vi "Write WriteUrgent.vi"(8 "error in (no error)":errorcluster, 10 "WriteUrgent":refnum<notifier>, 11 "ICPCON ET Data Model in":refnum<class "ICPCON ET Data Model.lvclass">) -> (0 "error out":errorcluster, 3 "ICPCON ET Data Model out":refnum<class "ICPCON ET Data Model.lvclass">)   [LabVIEW 2021, in "ICPCON ET Data Model.lvclass"]
uses:
  ICPCON ET Data Model.lvclass
  ICPCON ET Data Model.lvclass/ICPCON ET Data Model.ctl
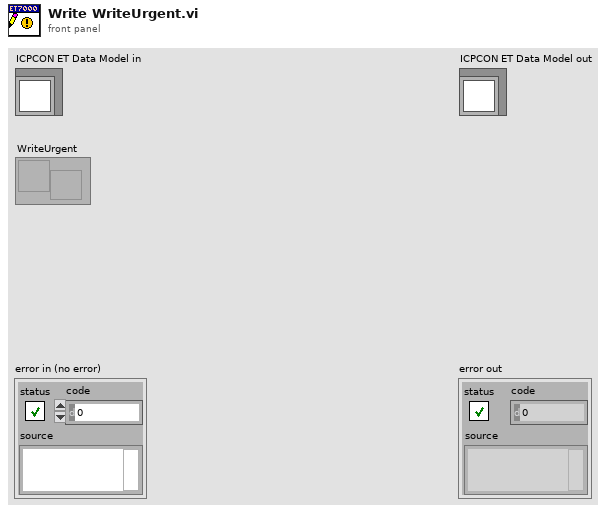
[diagram p1: front panel]
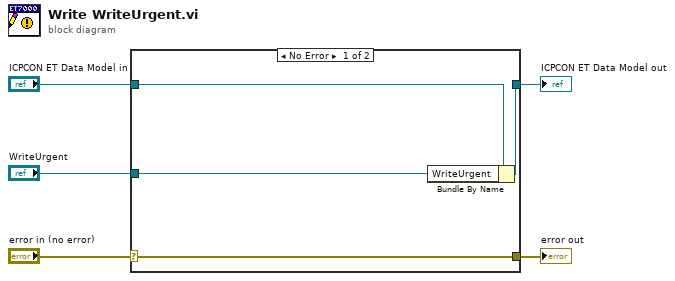
[diagram p0: block diagram]
diagram:
  n1 = case shown="No Error" "error in (no error)" {
    selector: "error in (no error)" -> [w9 w10]
    tunnel: [w9 w10] -> w4
    tunnel: [w7 w11] -> w2
    tunnel: "ICPCON ET Data Model in" -> [w8 w11]
    tunnel: "WriteUrgent" -> [w6 _]
    frame No Error {
      n2 = Bundle By Name(cluster=w8, "WriteUrgent"=w6) -> (w7:refnum<class "ICPCON ET Data Model.lvclass">)
    }
    frame Error {
    }
  }
  "error out" <- w4
  "ICPCON ET Data Model out" <- w2
